vi "Configure Output Range and Manual Value.vi"(0 "VISA resource name":refnum<visa-resource-name>, 5 "Output (1:1)":u16(ring)=1 items=["1"=1, "2"=2, "3"=3, "4"=4], 7 "Range (0:Off)":u16(ring) items=["Off", "Range 1 (On)", "Range 2", "Range 3", "Range 4", "Range 5"], 9 "Manual Output (0.00 %)":dbl format="%.2f", 11 "error in (no error)":errorcluster) -> (4 "VISA resource name out":refnum<visa-resource-name>, 15 "error out":errorcluster)   [LabVIEW 2010, in "Lake Shore 350.lvlib"]
doc: "Configures the Range and Manual Output Value for the Heater Outputs and the Unpowered Analog Outputs."
uses:
  <instrlib>/Lake Shore 350/Lake Shore 350.lvlib
  Instance           1 47Saved   Configure Output Range and Manual Value .vi
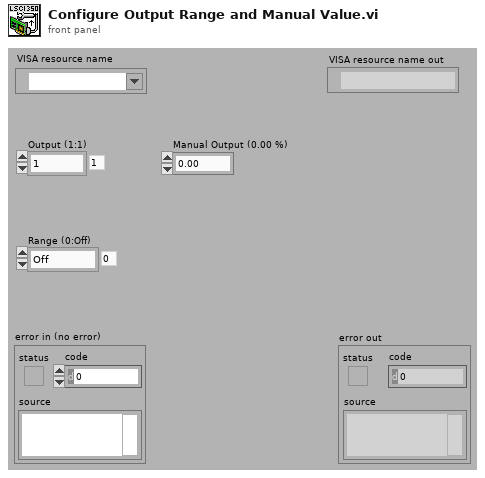
[diagram p1: front panel]
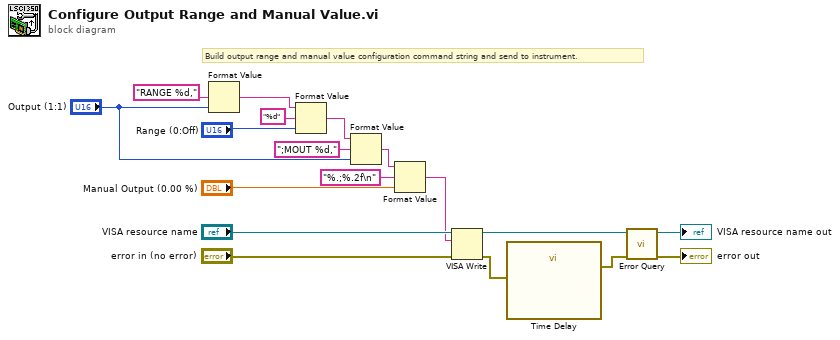
[diagram p0: block diagram]
diagram:
  # "Build output range and manual value configuration command string and send to instrument."
  n1 = Format Value(format string="RANGE %d,", value (0)="Output (1:1)") -> (output string=w4:string)  [unwired: 1 in]
  n2 = Format Value(string ("")=w4, format string="%d", value (0)="Range (0:Off)") -> (output string=w3:string)
  n3 = Format Value(string ("")=w3, format string=";MOUT %d,", value (0)="Output (1:1)") -> (output string=w2:string)
  n4 = Format Value(string ("")=w2, format string="%.;%.2f\n", value (0)="Manual Output (0.00 %)") -> (output string=w7:string)
  n5 = VISA Write(VISA resource name="VISA resource name", write buffer=w7, error in (no error)="error in (no error)") -> (VISA resource name out=w16:refnum<visa-resource-name>, error out=w13:errorcluster)  [unwired: 1 out]
  n6 = call "Time Delay"("error in (no error)"=w13) -> ("error out"=w12:errorcluster)  [unwired: 10 in]
  n7 = call <instrlib>:"Error Query.vi"("error in (no error)"=w12, "VISA resource name"=w16) -> ("error out"=→"error out":errorcluster, "VISA resource name out"=→"VISA resource name out":refnum<visa-resource-name>)  [unwired: 7 in, 1 out]
